vi "PID Command.vi"(0 "PulseVoltage":dbl, 1 "TCP from Orchid in":refnum<k5>, 3 "Starting index":bool, 4 "Measurement Type":enum32{"Volt", "SA"}(radio), 5 "적정 PRF":dbl, 7 "VTxIndex":i8, 9 "Target temp":dbl, 11 "Probe temp":dbl, 13 "tcp time out":dbl, 14 "Control enable":bool) -> (6 "PRF":dbl)   [LabVIEW 2016]
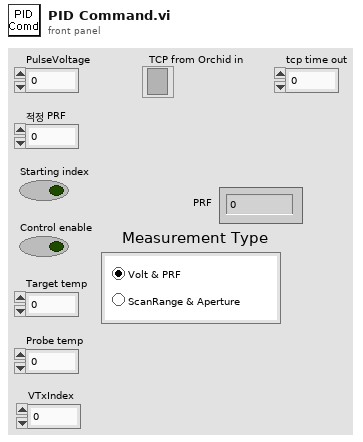
[diagram p1: front panel]
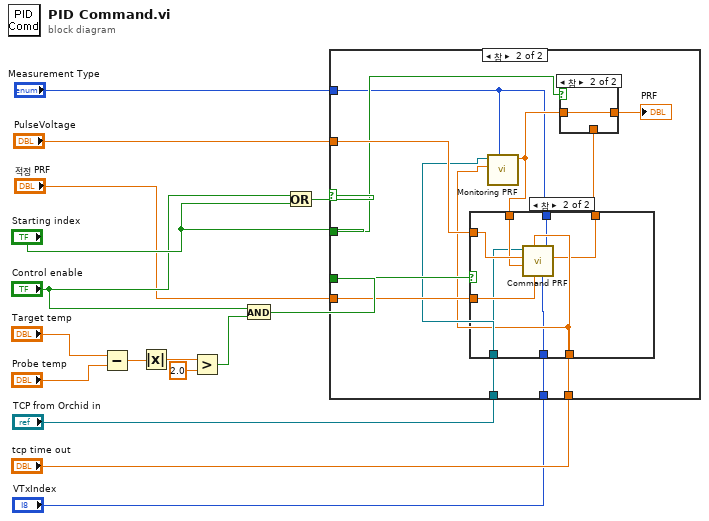
[diagram p0: block diagram]
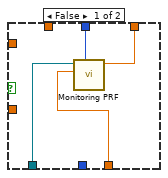
[diagram p4: hidden frame]
diagram:
  n1 = Subtract(x="Target temp", y="Probe temp") -> (x-y=w11:dbl)
  n2 = Absolute Value(x=w11) -> (abs(x)=w10:dbl)
  n3 = Greater?(x=w10, y=2.0) -> (0:w9:bool)
  n4 = And(x="Control enable", y=w9) -> (x .and. y?=w14:bool)
  n5 = Or(x="Control enable", y="Starting index") -> (x .or. y?=w15:bool)
  n6 = case shown="참" w15 {
    tunnel: "TCP from Orchid in" -> [_ w24]
    tunnel: "tcp time out" -> [_ w23]
    tunnel: "적정 PRF" -> [_ w27]
    tunnel: w14 -> [_ w26]
    tunnel: "PulseVoltage" -> [_ w25]
    tunnel: "Starting index" -> [_ w22]
    tunnel: "Measurement Type" -> [_ w18]
    tunnel: "VTxIndex" -> [_ w17]
    frame False {
    }
    frame True {
      n7 = call "Monitoring PRF.vi"("Measurement Type"=w18, "timeout (ms)"=w23, "TCP from Orchid in"=w24) -> ("PRF"=w21:dbl)  [unwired: 6 in, 1 out]
      n8 = case shown="참" w26 {
        tunnel: w24 -> [w33 w37]
        tunnel: w23 -> [w32 w39]
        tunnel: w27 -> [_ w38]
        tunnel: w25 -> [_ w41]
        tunnel: w21 -> [_ w40]
        tunnel: [w31 w36] -> w20
        tunnel: w18 -> [w30 w35]
        tunnel: w17 -> [_ w34]
        frame False {
          n9 = call "Monitoring PRF.vi"("Measurement Type"=w30, "timeout (ms)"=w32, "TCP from Orchid in"=w33) -> ("PRF"=w31:dbl)  [unwired: 6 in, 1 out]
        }
        frame True {
          n10 = call "Command PRF.vi"("VTxIndex"=w34, "Measurement Type"=w35, "PID PRF"=w38, "timeout (ms)"=w39, "Previous PRF"=w40, "Voltage"=w41, "TCP from Orchid in"=w37) -> ("PRF"=w36:dbl)  [unwired: 3 in, 1 out]
        }
      }
      n11 = case shown="참" w22 {
        tunnel: [w28 w29] -> w19
        tunnel: w21 -> [_ w29]
        tunnel: w20 -> [w28 _]
        frame False {
        }
        frame True {
        }
      }
      "PRF" <- w19
    }
  }
